vi "get_ai_type_dictionary.vi"(8 "error in (no error)":errorcluster) -> (0 "error out":errorcluster, 2 "AI type dictionary":variant)   [LabVIEW 2018]
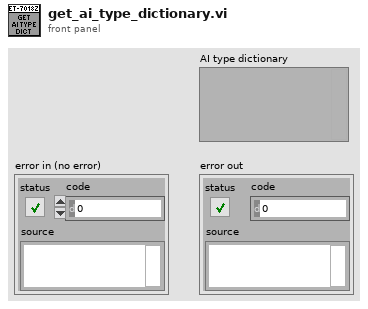
[diagram p1: front panel]
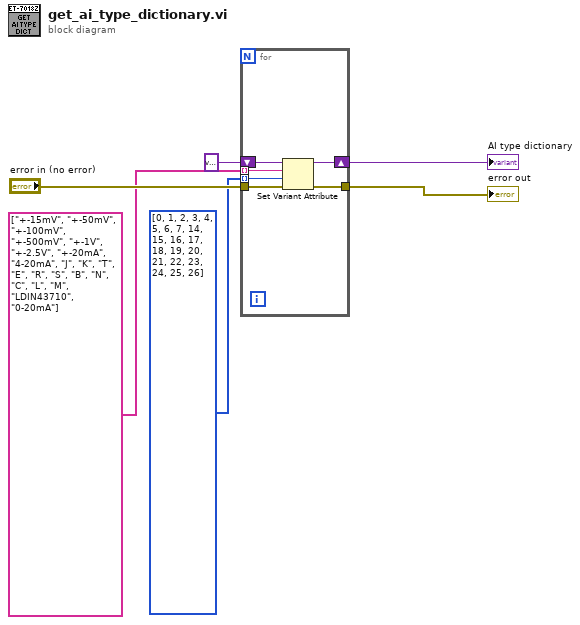
[diagram p0: block diagram]
diagram:
  n1 = for {
    shift-right: [w12] -> w4
    shift-left: variant ("variant") -> [w11]
    tunnel: string[] ["+-15mV", "+-50mV", "+-100mV", "+-500mV", "+-1V", "+-2.5V", "+-20mA", "4-20mA", "J", "K", "T", "E", "R", "S", "B", "N", "C", "L", "M", "LDIN43710", "0-20mA"] -> [w10] mode=indexing
    tunnel: u16[] [0, 1, 2, 3, 4, 5, 6, 7, 14, 15, 16, 17, 18, 19, 20, 21, 22, 23, 24, 25, 26] -> [w9] mode=indexing
    tunnel: "error in (no error)" -> [w8]
    tunnel: [w7] -> w5
    n2 = Set Variant Attribute(Variant=w11, name=w10, value=w9, error in=w8) -> (Variant out=w12:variant, error out=w7:errorcluster)  [unwired: 1 out]
  }
  "AI type dictionary" <- w4
  "error out" <- w5
